vi "getImage_action.vi"(0 "HGF_ImaqDx":refnum<class "HGF_ImaqDx.lvclass">, 2 "Image In":T1, 3 "Buffer Number":u32, 4 "Timeout (1000ms)":i32=1000, 5 "error in (no error)":errorcluster, 6 "Region of Interest":i32[](array[numeric]), 8 "Buffer Number Mode (Next)":T2) -> (11 "Frame Numbers":i32[](array[numeric]), 13 "Image Array":T1[](array[typedef]), 14 "dup HGF_ImaqDx":refnum<class "HGF_ImaqDx.lvclass">, 16 "Image Out":T1, 17 "Buffer Number Copied":i32, 18 "Buffer Index Copied":i32, 19 "error out":errorcluster)   [LabVIEW 2014, in "HGF_IMAQ.lvlib" / "HGF_ImaqDx.lvclass"]
doc: "Returns a copy of an acquired image. IMAQ Copy Acquired Buffer allows you to copy an image from onboard memory to system memory, or from driver-allocated system memory to user-allocated system memory.\n\nCall this VI only after calling IMAQdx Configure Acquisition.vi. If the image type does not match the video format of the camera, this VI changes the image type to a suitable format, at least for IMAQdx."
uses:
  HGF_ImaqDx.lvclass
  <resource>/objmgr/imaqdx.rc
  <vilib>/vision/Image Controls.llb/IMAQ Image.ctl
  <vilib>/vision/driver/IMAQdx.llb/IMAQdx Buffer Number Mode.ctl
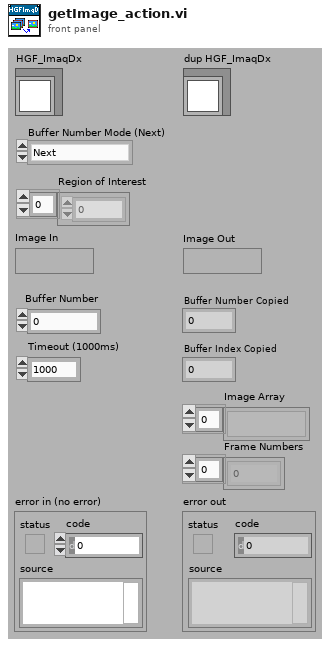
[diagram p1: front panel]
types:
  T1 = typedef "IMAQ Image.ctl" = refnum<image>
  T2 = typedef "NI_Vision_Acquisition_Software.lvlib/IMAQdx Buffer Number Mode.ctl" = enum32{"Next", "Last", "Buffer Number"}
  T3 = typedef "IMAQdx.ctl" = refnum<k21>
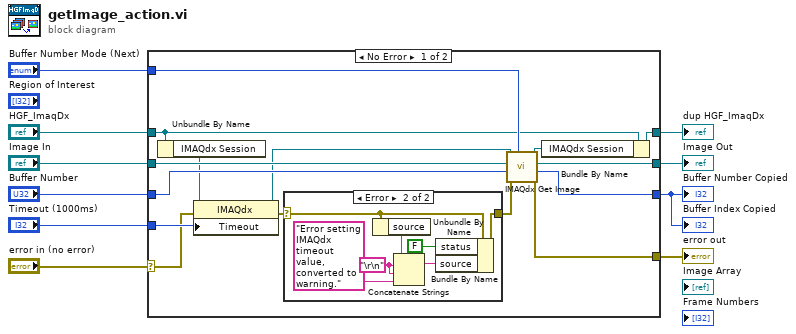
[diagram p0: block diagram]
diagram:
  n1 = case shown="No Error" "error in (no error)" {
    selector: "error in (no error)" -> [w13 w34]
    tunnel: "Image In" -> [w25 w35]
    tunnel: [w24 w35] -> w9
    tunnel: "Buffer Number Mode (Next)" -> [w23 _]
    tunnel: "Buffer Number" -> [w22 _]
    tunnel: [w21 _] -> w1
    tunnel: "HGF_ImaqDx" -> [w20 w36]
    tunnel: [w19 w36] -> w5
    tunnel: "Timeout (1000ms)" -> [w18 _]
    tunnel: [w16 w34] -> w3
    frame No Error {
      n2 = Unbundle By Name(w20) -> ("IMAQdx Session"=w14:T3)
      n3 = property class="IMAQdx"(reference=w14, error in=w13, "Timeout"=w18) -> (reference out=w17:T3, error out=w11:errorcluster)
      n4 = case shown="Error" w11 {
        selector: w11 -> [w26 w30]
        tunnel: [w26 w32] -> w12
        frame No Error {
        }
        frame Error {
          w27 = "\r\n"
          n5 = Unbundle By Name(w30) -> ("source"=w29:string)
          n6 = Concatenate Strings(w29, w27, w27, "Error setting IMAQdx timeout value, converted to warning." ("string")) -> (w31:string)
          n7 = Bundle By Name(cluster=w30, "status"=FALSE, "source"=w31) -> (w32:errorcluster)
        }
      }
      n8 = call <vilib>:"IMAQdx Get Image.vi"("Buffer Number Mode (Next)"=w23, "error in"=w12, "Buffer Number In"=w22, "Image In"=w25, "Session In"=w17) -> ("error out"=w16:errorcluster, "Buffer Number Out"=w21:u32, "Image Out"=w24:T1, "Session Out"=w15:T3)  [unwired: 3 out]
      n9 = Bundle By Name(cluster=w20, "IMAQdx Session"=w15) -> (w19:refnum<class "HGF_ImaqDx.lvclass">)
    }
    frame Error {
    }
  }
  "error out" <- w3
  "dup HGF_ImaqDx" <- w5
  "Buffer Number Copied" <- w1
  "Buffer Index Copied" <- w1
  "Image Out" <- w9
